vi "main 0.1.vi"() -> ()   [LabVIEW 2012]
panel:
  out "Waveform Chart":dbl(graph)
  out "sum":dbl
  in  "dark":bool
  in  "dark imgs":i32
  in  "dark?":bool
  in  "threshold":i32=1
  in  "avg[t] acc[f]":bool
  in  "avgs":i32=1
  out "img":dbl[][](graph)
  in  "exp time":dbl=0.01
  in  "binning":dbl=4.0
  in  "close":bool
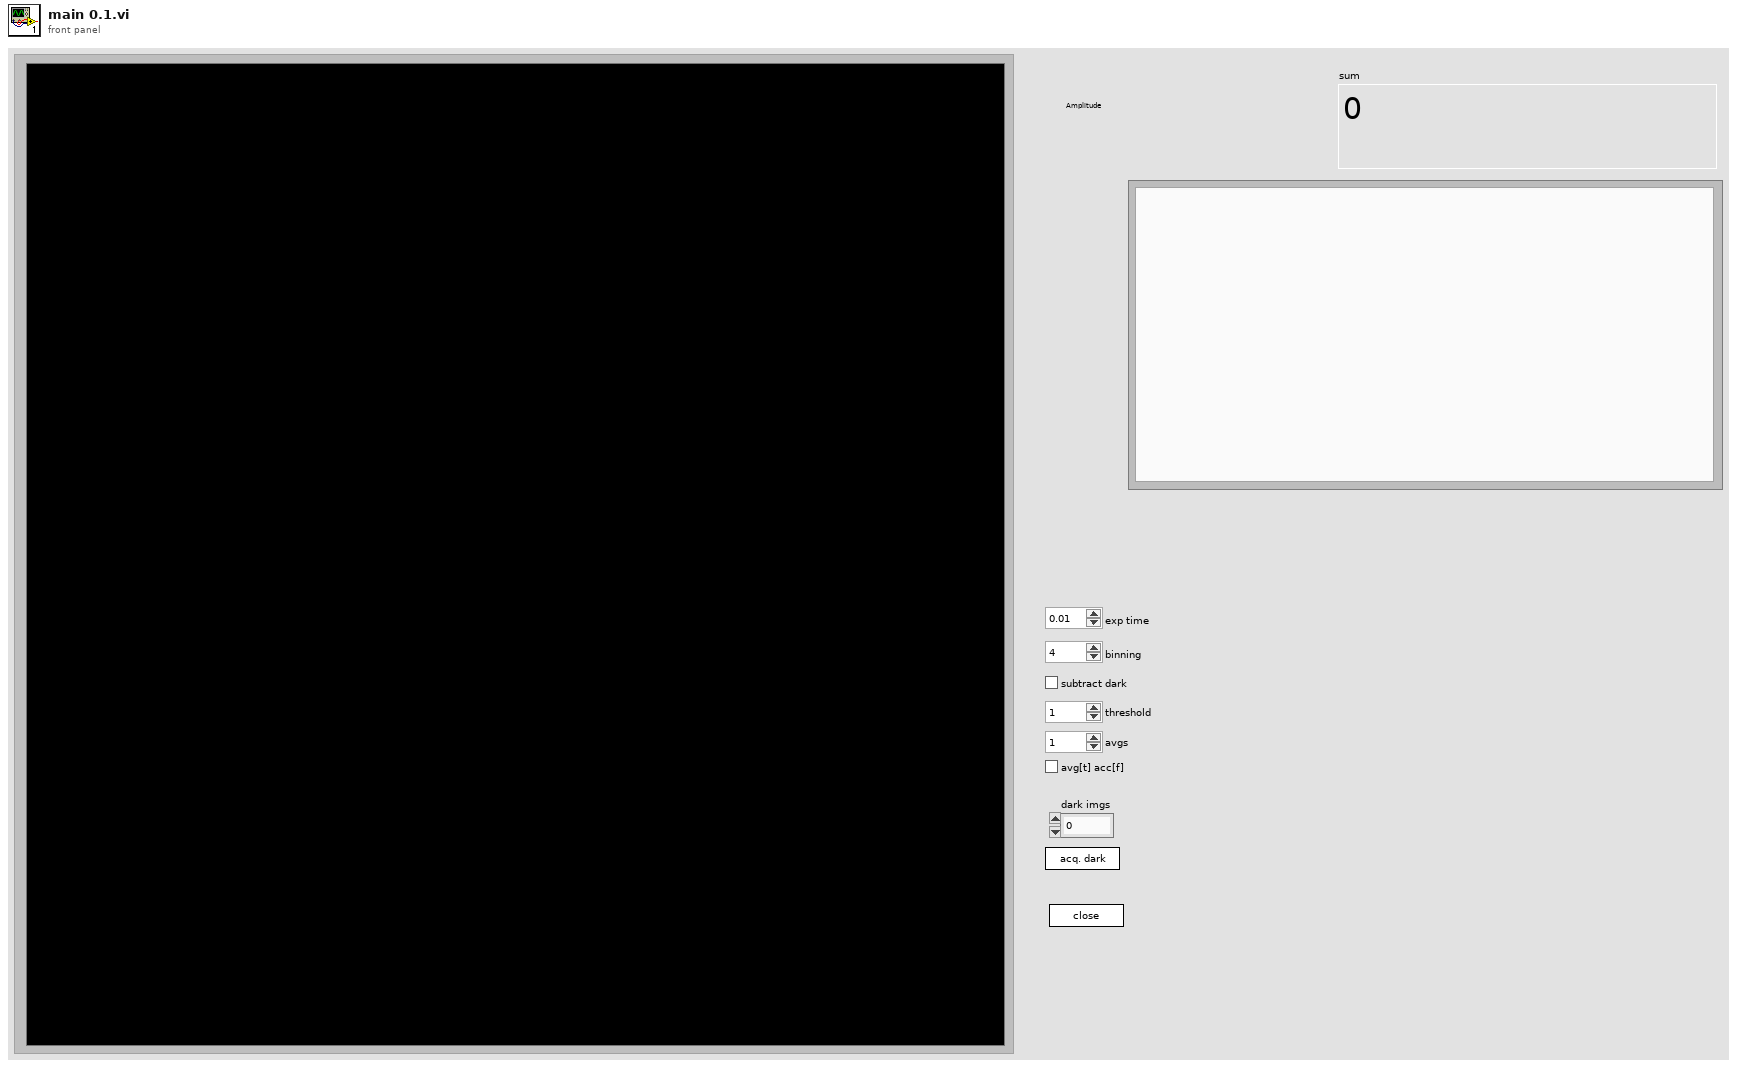
[diagram p1: front panel]
types:
  T1 = cluster{"height":u32, "width":u32, "datatype":u32}
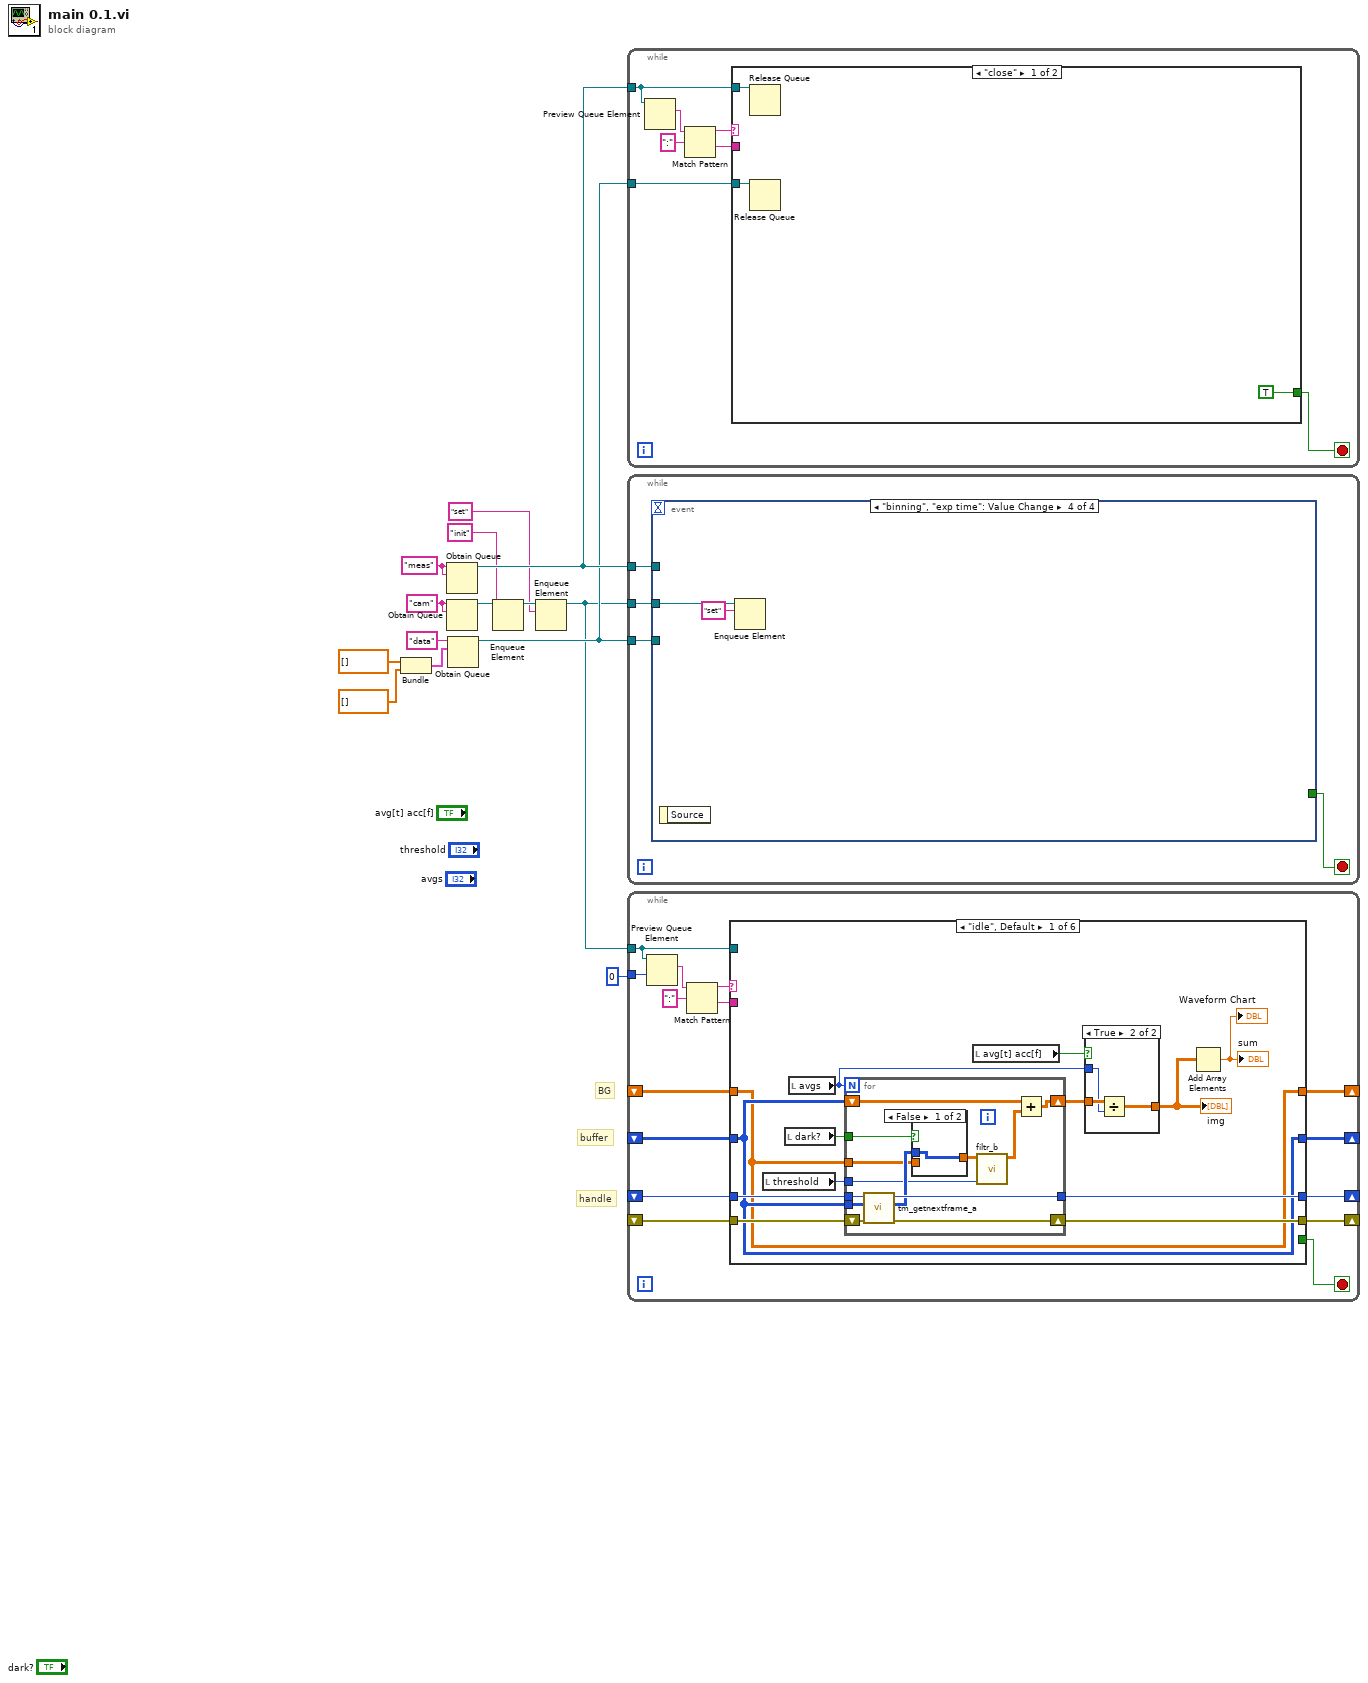
[diagram p0: block diagram]
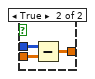
[diagram p4: hidden frame]
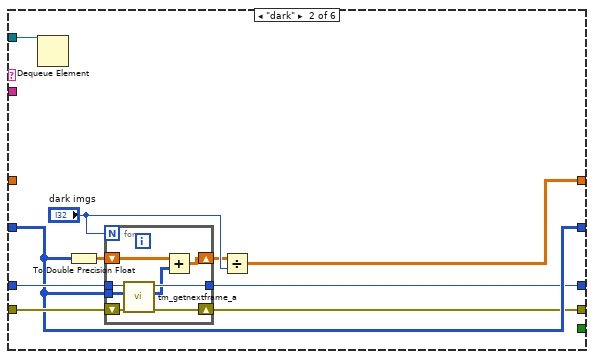
[diagram p5: hidden frame]
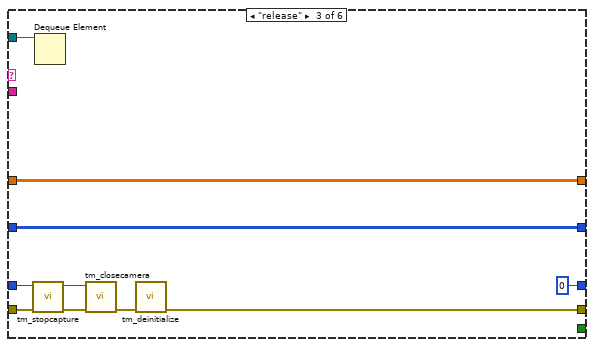
[diagram p6: hidden frame]
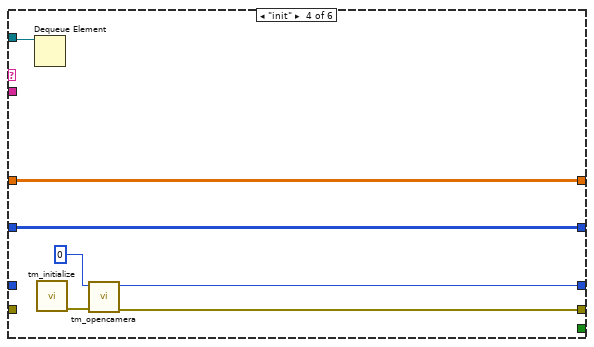
[diagram p7: hidden frame]
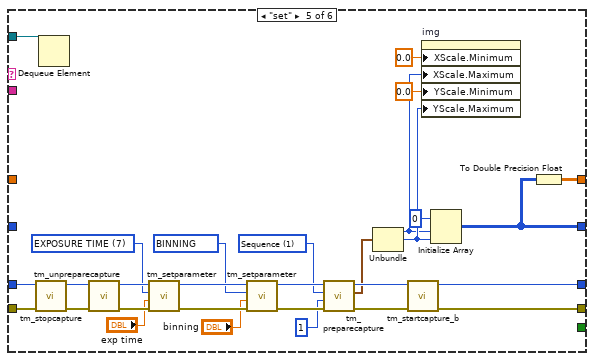
[diagram p8: hidden frame]
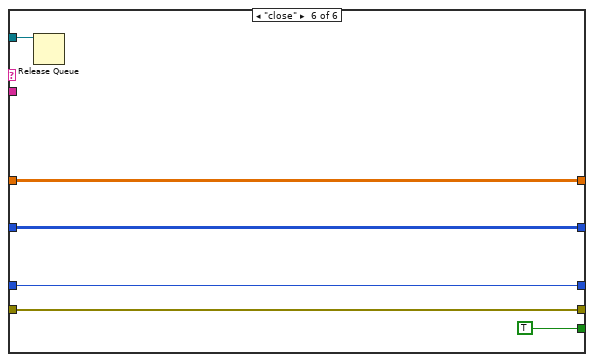
[diagram p9: hidden frame]
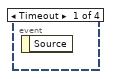
[diagram p10: hidden frame]
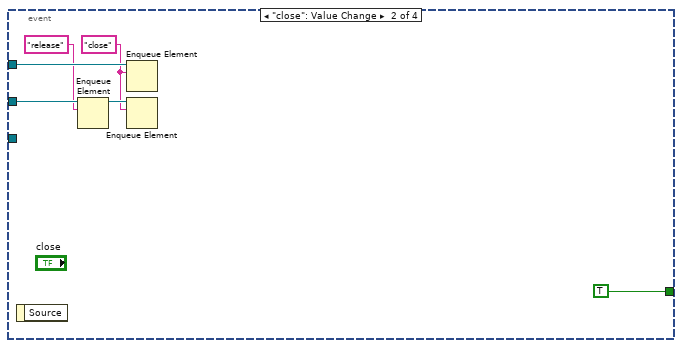
[diagram p11: hidden frame]
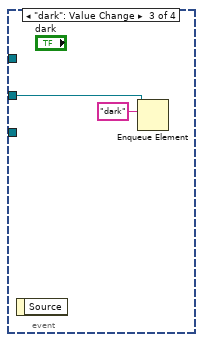
[diagram p12: hidden frame]
diagram:
  w9 = "meas" ("name (unnamed)")
  w12 = "cam" ("name (unnamed)")
  # "BG"
  # "handle"
  # "buffer"
  n1 = Bundle(dbl[] [], dbl[] []) -> (w10:cluster{dbl[], dbl[]})  [unwired: 1 in]
  n2 = Obtain Queue(name (unnamed)=w9, element data type=w9) -> (queue out=w7:refnum<queue>)  [unwired: 3 in, 2 out]
  n3 = Obtain Queue(name (unnamed)=w12, element data type=w12) -> (queue out=w14:refnum<queue>)  [unwired: 3 in, 2 out]
  n4 = Obtain Queue(name (unnamed)="data", element data type=w10) -> (queue out=w6:refnum<queue>)  [unwired: 3 in, 2 out]
  n5 = Enqueue Element(queue=w14, element="init") -> (queue out=w4:refnum<queue>)  [unwired: 2 in, 2 out]
  n6 = Enqueue Element(queue=w4, element="set") -> (queue out=w3:refnum<queue>)  [unwired: 2 in, 2 out]
  n7 = while {
    tunnel: w7 -> [w17]
    tunnel: w6 -> [w16]
    stop <- w15 stop-if-true
    n8 = Preview Queue Element(queue=w17) -> (element=w21:string)  [unwired: 2 in, 3 out]
    n9 = Match Pattern(string=w21, regular expression=":") -> (before substring=w19:string, after substring=w18:string)  [unwired: 1 in, 2 out]
    n10 = case shown="\"close\"" w19 {
      tunnel: w18 -> [_ _]
      tunnel: w17 -> [w23 _]
      tunnel: w16 -> [w24 _]
      tunnel: [TRUE _] -> w15
      frame "close" {
        n11 = Release Queue(queue=w23) -> ()  [unwired: 2 in, 3 out]
        n12 = Release Queue(queue=w24) -> ()  [unwired: 2 in, 3 out]
      }
      frame "idle", Default {
      }
    }
  }
  n13 = while {
    tunnel: w3 -> [w28]
    tunnel: w7 -> [w27]
    tunnel: w6 -> [w26]
    stop <- w25 stop-if-true
    n14 = event shown="[3] \"binning\", \"exp time\": Value Change" {
      selector: _ -> [_ _ _ _]
      dyn-events: _ -> [_ _ _ _]
      timeout: _ -> [_ _ _ _]
      tunnel: w28 -> [_ w33 w36 w38]
      tunnel: w27 -> [_ w34 _ _]
      tunnel: w26 -> [_ _ _ _]
      tunnel: [_ TRUE _ _] -> w25
      event Timeout {
        n15 = event-data() -> ()  [unwired: 1 in, 1 out]
      }
      event "close": Value Change {
        w30 = "close" ("element")
        n16 = event-data() -> ()  [unwired: 1 in, 1 out]
        n17 = Enqueue Element(queue=w33, element="release") -> (queue out=w32:refnum<queue>)  [unwired: 2 in, 2 out]
        n18 = Enqueue Element(queue=w34, element=w30) -> ()  [unwired: 2 in, 3 out]
        n19 = Enqueue Element(queue=w32, element=w30) -> ()  [unwired: 2 in, 3 out]
      }
      event "dark": Value Change {
        n20 = event-data() -> ()  [unwired: 1 in, 1 out]
        n21 = Enqueue Element(queue=w36, element="dark") -> ()  [unwired: 2 in, 3 out]
      }
      event "binning", "exp time": Value Change {
        n22 = event-data() -> ()  [unwired: 1 in, 1 out]
        n23 = Enqueue Element(queue=w38, element="set") -> ()  [unwired: 2 in, 3 out]
      }
    }
  }
  n24 = while {
    tunnel: w3 -> [w49]
    shift-right: [w47] -> _
    shift-left: _ -> [w46]
    shift-right: [w45] -> _
    shift-left: _ -> [w44]
    shift-right: [w43] -> _
    shift-left: _ -> [w42]
    shift-right: [w41] -> _
    shift-left: _ -> [w40]
    tunnel: 0 -> [w39]
    stop <- w48 stop-if-true
    n25 = Preview Queue Element(queue=w49, timeout in ms (-1)=w39) -> (element=w53:string)  [unwired: 1 in, 3 out]
    n26 = Match Pattern(string=w53, regular expression=":") -> (before substring=w51:string, after substring=w50:string)  [unwired: 1 in, 2 out]
    n27 = case shown="\"idle\", Default" w51 {
      tunnel: w50 -> [_ _ _ _ _ _]
      tunnel: w49 -> [_ w97 w115 w116 w128 w157]
      tunnel: [_ _ _ _ _ TRUE] -> w48
      tunnel: [w61 w88 w107 w121 w129 w152] -> w47
      tunnel: w46 -> [w63 w94 w111 _ w151 w152]
      tunnel: [w62 w89 u32 0 ("Handle out") w119 w130 w153] -> w45
      tunnel: w44 -> [w64 w93 w112 _ w149 w153]
      tunnel: [w57 w90 w113 w117 w131 w154] -> w43
      tunnel: w42 -> [w57 w90 w113 w117 _ w154]
      tunnel: [w56 w91 w114 w118 w132 w155] -> w41
      tunnel: w40 -> [w56 _ w114 w118 _ w155]
      frame "idle", Default {
        n28 = local read "threshold"() -> (w65:i32)
        n29 = local read "dark?"() -> (w66:bool)
        n30 = local read "avgs"() -> (w58:i32)
        n31 = for {
          N: w58 -> [_]
          tunnel: w66 -> [w83]
          tunnel: w57 -> [w81]
          tunnel: w64 -> [w82]
          tunnel: w65 -> [w75]
          tunnel: [w79] -> w62
          shift-right: [w78] -> w61
          shift-left: w63 -> [w80]
          tunnel: w56 -> [w74]
          shift-right: [w71] -> w59
          shift-left: w57 -> [w73]
          n32 = call "tm_getnextframe_a.vi"("error in (no error)"=w80, "Buffer"=w81, "Handle in"=w82) -> ("error out"=w78:errorcluster, "Data"=w77:u16[][], "Handle out"=w79:u32)  [unwired: 6 in]
          n33 = case shown="False" w83 {
            tunnel: [w84 w87] -> w76
            tunnel: w77 -> [w84 w86]
            tunnel: w74 -> [_ w85]
            frame False {
            }
            frame True {
              n34 = Subtract(x=w86, y=w85) -> (x-y=w87:dbl[][])
            }
          }
          n35 = call "filtr_b.vi"("threshold"=w75, "input array"=w76) -> ("output array"=w72:dbl[][])  [unwired: 9 in]
          n36 = Add(x=w73, y=w72) -> (x+y=w71:dbl[][])
        }
        n37 = local read "avg[t] acc[f]"() -> (w60:bool)
        n38 = case shown="True" w60 {
          tunnel: w59 -> [w67 w70]
          tunnel: w58 -> [_ w69]
          tunnel: [w67 w68] -> w55
          frame False {
          }
          frame True {
            n39 = Divide(x=w70, y=w69) -> (x/y=w68:dbl[][])
          }
        }
        "img" <- w55
        n40 = Add Array Elements(numeric array=w55) -> (sum=→"sum" →"Waveform Chart":dbl)
      }
      frame "dark" {
        n41 = Dequeue Element(queue=w97) -> ()  [unwired: 2 in, 4 out]
        n42 = To Double Precision Float(number=w90) -> (double precision float=w92:dbl[][])
        n43 = for {
          N: "dark imgs" -> [_]
          tunnel: [w104] -> w89
          shift-right: [w103] -> w88
          shift-left: w94 -> [w105]
          shift-right: [w101] -> w95
          shift-left: w92 -> [w102]
          tunnel: w93 -> [w99]
          tunnel: w90 -> [w98]
          n44 = call "tm_getnextframe_a.vi"("error in (no error)"=w105, "Buffer"=w98, "Handle in"=w99) -> ("error out"=w103:errorcluster, "Data"=w100:u16[][], "Handle out"=w104:u32)  [unwired: 6 in]
          n45 = Add(x=w102, y=w100) -> (x+y=w101:dbl[][])
        }
        n46 = Divide(x=w95, y="dark imgs") -> (x/y=w91:dbl[][])
      }
      frame "release" {
        n47 = call "tm_stopcapture.vi"("error in (no error)"=w111, "Handle in"=w112) -> ("error out"=w109:errorcluster, "Handle out"=w110:u32)  [unwired: 8 in]
        n48 = Dequeue Element(queue=w115) -> ()  [unwired: 2 in, 4 out]
        n49 = call "tm_closecamera.vi"("error in (no error)"=w109, "Handle in"=w110) -> ("error out"=w108:errorcluster)  [unwired: 9 in]
        n50 = call "tm_deinitialize.vi"("error in (no error)"=w108) -> ("error out"=w107:errorcluster)  [unwired: 10 in]
      }
      frame "init" {
        n51 = Dequeue Element(queue=w116) -> ()  [unwired: 2 in, 4 out]
        n52 = call "tm_initialize.vi"() -> ("error out"=w122:errorcluster)  [unwired: 8 in, 3 out]
        n53 = call "tm_opencamera.vi"("error in (no error)"=w122, "Camera Index"=u32 0) -> ("error out"=w121:errorcluster, "Handle out"=w119:u32)  [unwired: 7 in, 1 out]
      }
      frame "set" {
        w137 = 1 items=["Snap", "Sequence"] ("Capture mode")
        w141 = u32 4215968 items=["BINNING"=4215968, "BITS PER CHANNEL"=2, "ACTIVE VIEW INDEX"=3, "CCD MODE"=4, "SENSOR MODE"=5, "READOUT MODE"=6, "EXPOSURE TIME"=7, "CONTRAST GAIN"=8, "CONTRAST OFFSET"=9, "LIGHT MODE"=10, "SENSITIVITY"=11, "WHITE BALANCE"=12, "PHOTON IMAGING MODE"=13, "HIGH DYNAMIC RANGE MODE"=14, "TRIGGER SOURCE"=15, "TRIGGER ACTIVE"=16, "TRIGGER MODE"=17, "TRIGGER POLARITY"=18, "TRIGGER GLOBAL EXPOSURE"=19, "FIRST TRIGGER BEHAVIOR"=20, "TRIGGER TIMES"=21, "OUTPUT TRIGGER POLARITY"=22, "OUTPUT TRIGGER DELAY"=23, "OUTPUT TRIGGER PERIOD"=24, "TEMPERATURE"=25, "TEMPERATURE TARGET"=26, "SENSOR COOLER FAN"=27, "MECHANICAL SHUTTER"=28, "BACK FOCUS POSITION"=29, "FRAMEBUNDLE MODE"=30, "FRAMEBUNDLE NUMBER"=31, "LINEBUNDLE HEIGHT"=32, "TRIGGER CONNECTOR"=33, "IMAGE PIXEL TYPE"=34, "OUTPUT TRIGGER KIND"=35, "READOUT DIRECTION"=36, "CHANNEL SYNC"=37] ("Parameter")
        w145 = u32 7 items=["BINNING"=4215968, "BITS PER CHANNEL"=2, "ACTIVE VIEW INDEX"=3, "CCD MODE"=4, "SENSOR MODE"=5, "READOUT MODE"=6, "EXPOSURE TIME"=7, "CONTRAST GAIN"=8, "CONTRAST OFFSET"=9, "LIGHT MODE"=10, "SENSITIVITY"=11, "WHITE BALANCE"=12, "PHOTON IMAGING MODE"=13, "HIGH DYNAMIC RANGE MODE"=14, "TRIGGER SOURCE"=15, "TRIGGER ACTIVE"=16, "TRIGGER MODE"=17, "TRIGGER POLARITY"=18, "TRIGGER GLOBAL EXPOSURE"=19, "FIRST TRIGGER BEHAVIOR"=20, "TRIGGER TIMES"=21, "OUTPUT TRIGGER POLARITY"=22, "OUTPUT TRIGGER DELAY"=23, "OUTPUT TRIGGER PERIOD"=24, "TEMPERATURE"=25, "TEMPERATURE TARGET"=26, "SENSOR COOLER FAN"=27, "MECHANICAL SHUTTER"=28, "BACK FOCUS POSITION"=29, "FRAMEBUNDLE MODE"=30, "FRAMEBUNDLE NUMBER"=31, "LINEBUNDLE HEIGHT"=32, "TRIGGER CONNECTOR"=33, "IMAGE PIXEL TYPE"=34, "OUTPUT TRIGGER KIND"=35, "READOUT DIRECTION"=36, "CHANNEL SYNC"=37] ("Parameter")
        n54 = call "tm_stopcapture.vi"("error in (no error)"=w151, "Handle in"=w149) -> ("error out"=w150:errorcluster, "Handle out"=w148:u32)  [unwired: 8 in]
        n55 = Dequeue Element(queue=w128) -> ()  [unwired: 2 in, 4 out]
        n56 = call "tm_unpreparecapture.vi"("error in (no error)"=w150, "Handle in"=w148) -> ("error out"=w147:errorcluster, "Handle out"=w146:u32)  [unwired: 8 in]
        n57 = call "tm_setparameter.vi"("error in (no error)"=w147, "Value in"="exp time", "Parameter"=w145, "Handle in"=w146) -> ("error out"=w142:errorcluster, "Handle out"=w143:u32)  [unwired: 6 in]
        n58 = call "tm_setparameter.vi"("error in (no error)"=w142, "Value in"="binning", "Parameter"=w141, "Handle in"=w143) -> ("error out"=w138:errorcluster, "Handle out"=w139:u32)  [unwired: 6 in]
        n59 = call "tm_preparecapture.vi"("error in (no error)"=w138, "Frames"=1, "Capture mode"=w137, "Handle in"=w139) -> ("error out"=w134:errorcluster, "Buffer Info"=w133:T1, "Handle out"=w135:u32)  [unwired: 4 in, 1 out]
        n60 = Unbundle(w133) -> ("height"=w126:u32, "width"=w127:u32)  [unwired: 1 out]
        n61 = call "tm_startcapture_b.vi"("error in (no error)"=w134, "Handle in"=w135) -> ("error out"=w129:errorcluster, "Handle out"=w130:u32)  [unwired: 8 in]
        n62 = property on="img" class="IntGraph (strict)"("XScale.Minimum"=0.0 ("X Scale.Range:Minimum"), "XScale.Maximum"=w126, "YScale.Minimum"=0.0 ("Y Scale.Range:Minimum"), "YScale.Maximum"=w127) -> ()  [unwired: 2 in, 2 out]
        n63 = Initialize Array(u16 0 ("element"), w126, w127) -> (w131:u16[][])
        n64 = To Double Precision Float(number=w131) -> (double precision float=w132:dbl[][])
      }
      frame "close" {
        n65 = Release Queue(queue=w157) -> ()  [unwired: 2 in, 3 out]
      }
    }
  }
